vi "COMI PG Start.vi"(7 "num_pulses":u32, 9 "freq":dbl, 10 "ch":i32, 11 "hDevice":u32) -> (2 "function return":dbl, 3 "hDevice out":u32)   [LabVIEW 2017, in "Comidll.lvlib"]
doc: "double (COMI_PG_Start) (HANDLE hDevice, int ch, double freq, unsigned int num_pulses);"
uses:
  <userlib>/Comidll/Comidll.lvlib
  <userlib>/Comidll/Comidll.dll
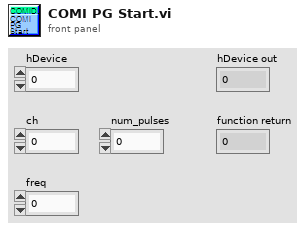
[diagram p1: front panel]
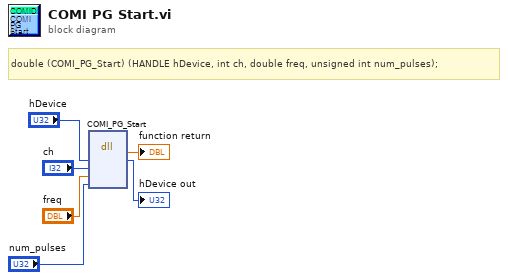
[diagram p0: block diagram]
diagram:
  # "double\t(COMI_PG_Start) (HANDLE hDevice, int ch, double freq, unsigned int num_pulses);"
  n1 = dll-call lib="C:/Program Files/National Instruments/LabVIEW 2017/user.lib/Comidll/Comidll.*" fn="COMI_PG_Start"("hDevice"="hDevice", "ch"="ch", "freq"="freq", "num_pulses"="num_pulses") -> (→"function return":dbl, "hDevice"=→"hDevice out":u32)  [unwired: 6 in, 2 out]
